vi "SCM2_T_Read_Remote.vi"() -> ()   [LabVIEW 2018]
panel:
  out "error out 4":errorcluster
  in  "stop":bool
  out "PROBE (K)":dbl=-17.9883723 format="%#_5g"
  out "error out 3":errorcluster
  out "3HE POT (K)":dbl=-17.9883723 format="%#_5g"
  out "error out 2":errorcluster
  out "1K POT (K)":dbl=-17.9883723 format="%#_5g"
  out "error out 1":errorcluster
  in  "port":u16=3376
  in  "error in (no error) 2":errorcluster
  in  "Data mac ip address":string="146.201.200.173"
  out "SORB (K)":dbl=-17.9883723 format="%#_5g"
  # "Note\n(1) Exception of the firewall should be configured.\n(2) With some (not all) connection with PC's, it is successful only when the VI is first executed. If the VI is stopped (normally or by aborting), \nthe subsequent connection is only possible with a new port number."
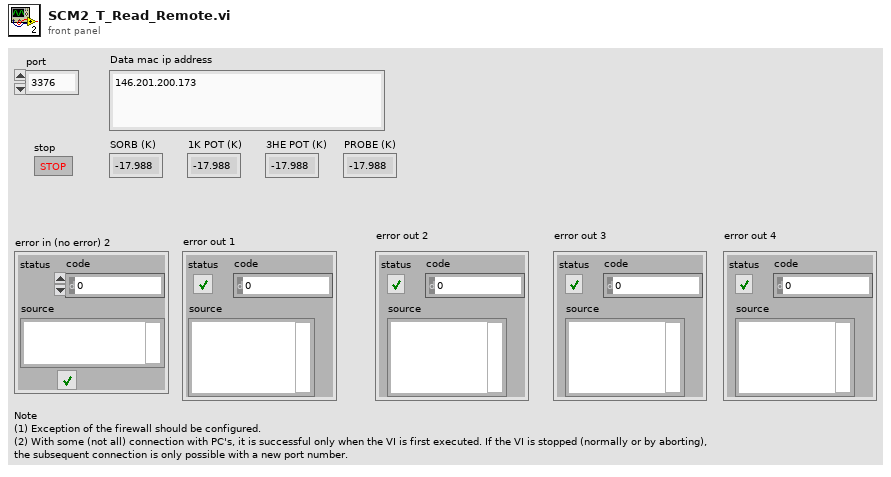
[diagram p1: front panel]
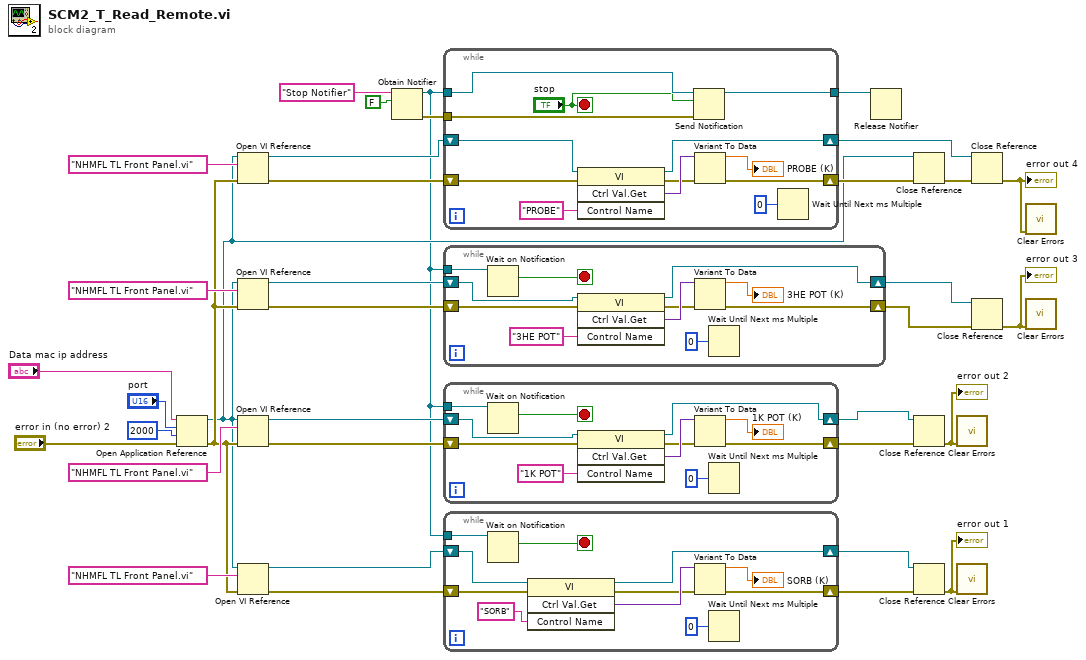
[diagram p0: block diagram]
diagram:
  n1 = Open Application Reference(8:"error in (no error) 2", 9:2000 ("timeout ms (60000)"), 10:"port", 11:"Data mac ip address") -> (0:w10:errorcluster, 3:w9:refnum<vi>)
  n2 = Open VI Reference(application reference (local)=w9, vi path="NHMFL TL Front Panel.vi" ("VI name"), error in (no error)=w10) -> (vi reference=w12:refnum<vi>, error out=w17:errorcluster)  [unwired: 3 in]
  n3 = Open VI Reference(application reference (local)=w9, vi path="NHMFL TL Front Panel.vi" ("VI name"), error in (no error)=w10) -> (vi reference=w19:refnum<vi>, error out=w22:errorcluster)  [unwired: 3 in]
  n4 = Open VI Reference(application reference (local)=w9, vi path="NHMFL TL Front Panel.vi" ("VI name"), error in (no error)=w10) -> (vi reference=w24:refnum<vi>, error out=w27:errorcluster)  [unwired: 3 in]
  n5 = Open VI Reference(application reference (local)=w9, vi path="NHMFL TL Front Panel.vi" ("VI name"), error in (no error)=w10) -> (vi reference=w29:refnum<vi>, error out=w33:errorcluster)  [unwired: 3 in]
  n6 = Obtain Notifier(name (unnamed)="Stop Notifier", notification data type=FALSE ("stop 2")) -> (notifier out=w5:refnum<notifier>, error out=w8:errorcluster)  [unwired: 2 in, 1 out]
  n7 = while {
    shift-right: [w47] -> w14
    shift-left: w12 -> [w48]
    shift-right: [w49] -> w16
    shift-left: w17 -> [w43]
    tunnel: w5 -> [w40]
    tunnel: w8 -> [w39]
    tunnel: [w37] -> w4
    stop <- "stop" stop-if-true
    n8 = invoke class="VI" method="Ctrl Val.Get"(reference=w48, error in=w43, "Control Name"="PROBE") -> (reference out=w47:refnum<vi>, error out=w45:errorcluster, "Get Control Value Variant"=w46:variant)  [unwired: 1 in, 1 out]
    n9 = Send Notification(notification="stop", notifier=w40, error in (no error)=w39) -> (notifier out=w37:refnum<notifier>)  [unwired: 1 out]
    n10 = Variant To Data(error in=w45, Variant=w46) -> (data=→"PROBE (K)":dbl, error out=w49:errorcluster)  [unwired: 1 in]
    n11 = Wait Until Next ms Multiple(millisecond multiple=u32 0) -> ()  [unwired: 1 out]
  }
  n12 = while {
    shift-right: [w58] -> w21
    shift-left: w19 -> [w59]
    shift-right: [w60] -> w1
    shift-left: w22 -> [w54]
    tunnel: w5 -> [w51]
    stop <- w50 stop-if-true
    n13 = Wait on Notification(notifier=w51) -> (notification=w50:bool)  [unwired: 3 in, 3 out]
    n14 = invoke class="VI" method="Ctrl Val.Get"(reference=w59, error in=w54, "Control Name"="3HE POT") -> (reference out=w58:refnum<vi>, error out=w56:errorcluster, "Get Control Value Variant"=w57:variant)  [unwired: 1 in, 1 out]
    n15 = Variant To Data(error in=w56, Variant=w57) -> (data=→"3HE POT (K)":dbl, error out=w60:errorcluster)  [unwired: 1 in]
    n16 = Wait Until Next ms Multiple(millisecond multiple=u32 0) -> ()  [unwired: 1 out]
  }
  n17 = while {
    shift-right: [w69] -> w26
    shift-left: w24 -> [w70]
    shift-right: [w71] -> w2
    shift-left: w27 -> [w65]
    tunnel: w5 -> [w62]
    stop <- w61 stop-if-true
    n18 = Wait on Notification(notifier=w62) -> (notification=w61:bool)  [unwired: 3 in, 3 out]
    n19 = invoke class="VI" method="Ctrl Val.Get"(reference=w70, error in=w65, "Control Name"="1K POT") -> (reference out=w69:refnum<vi>, error out=w67:errorcluster, "Get Control Value Variant"=w68:variant)  [unwired: 1 in, 1 out]
    n20 = Variant To Data(error in=w67, Variant=w68) -> (data=→"1K POT (K)":dbl, error out=w71:errorcluster)  [unwired: 1 in]
    n21 = Wait Until Next ms Multiple(millisecond multiple=u32 0) -> ()  [unwired: 1 out]
  }
  n22 = while {
    shift-right: [w80] -> w32
    shift-left: w29 -> [w81]
    shift-right: [w82] -> w3
    shift-left: w33 -> [w76]
    tunnel: w5 -> [w73]
    stop <- w72 stop-if-true
    n23 = Wait on Notification(notifier=w73) -> (notification=w72:bool)  [unwired: 3 in, 3 out]
    n24 = invoke class="VI" method="Ctrl Val.Get"(reference=w81, error in=w76, "Control Name"="SORB") -> (reference out=w80:refnum<vi>, error out=w78:errorcluster, "Get Control Value Variant"=w79:variant)  [unwired: 1 in, 1 out]
    n25 = Variant To Data(error in=w78, Variant=w79) -> (data=→"SORB (K)":dbl, error out=w82:errorcluster)  [unwired: 1 in]
    n26 = Wait Until Next ms Multiple(millisecond multiple=u32 0) -> ()  [unwired: 1 out]
  }
  n27 = Release Notifier(notifier=w4) -> ()  [unwired: 2 in, 3 out]
  n28 = Close Reference(reference=w9, error in (no error)=w16) -> (error out=w15:errorcluster)
  n29 = Close Reference(reference=w26, error in (no error)=w2) -> (error out=w23:errorcluster)
  "error out 2" <- w23
  n30 = Close Reference(reference=w32, error in (no error)=w3) -> (error out=w28:errorcluster)
  "error out 1" <- w28
  n31 = call <vilib>:"Clear Errors.vi"("error in (no error)"=w23) -> ()  [unwired: 5 in, 2 out]
  n32 = call <vilib>:"Clear Errors.vi"("error in (no error)"=w28) -> ()  [unwired: 5 in, 2 out]
  n33 = Close Reference(reference=w14, error in (no error)=w15) -> (error out=w11:errorcluster)
  "error out 4" <- w11
  n34 = Close Reference(reference=w21, error in (no error)=w1) -> (error out=w18:errorcluster)
  "error out 3" <- w18
  n35 = call <vilib>:"Clear Errors.vi"("error in (no error)"=w11) -> ()  [unwired: 5 in, 2 out]
  n36 = call <vilib>:"Clear Errors.vi"("error in (no error)"=w18) -> ()  [unwired: 5 in, 2 out]
